vi "cipher log.vi"() -> (8 "password to cipher log":string)   [LabVIEW 2012]
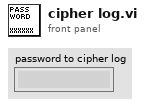
[diagram p1: front panel]
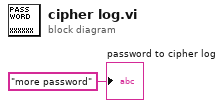
[diagram p0: block diagram]
diagram:
  "password to cipher log" <- "more password" ("password to cipher users")
